vi "UserInput-String.vi"() -> ()   [LabVIEW 2019]
panel:
  in  "Clear Form":bool
  in  "Copy String":bool
  out "String Indicator - Output":string
  in  "String Control - Input":string
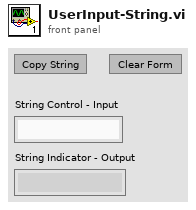
[diagram p1: front panel]
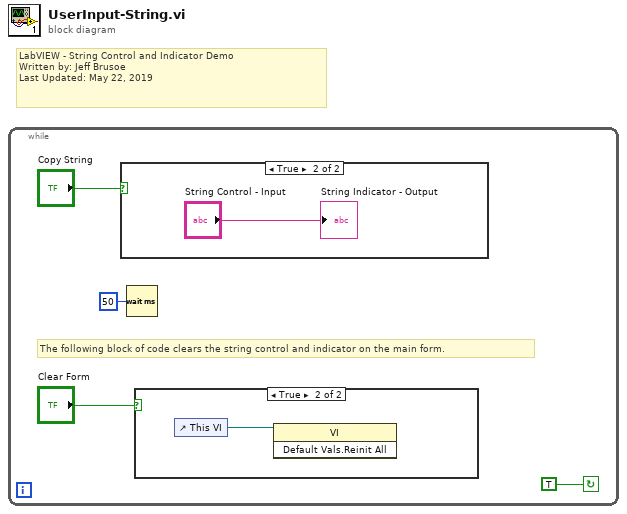
[diagram p0: block diagram]
diagram:
  # "LabVIEW - String Control and Indicator Demo\nWritten by: Jeff Brusoe\nLast Updated: May 22, 2019"
  n1 = while {
    stop <- TRUE continue-if-true
    # "The following block of code clears the string control and indicator on the main form."
    n2 = case shown="True" "Copy String" {
      frame False {
      }
      frame True {
        "String Indicator - Output" <- "String Control - Input"
      }
    }
    n3 = Wait (ms)(milliseconds to wait=u32 50) -> ()  [unwired: 1 out]
    n4 = case shown="True" "Clear Form" {
      frame False {
      }
      frame True {
        n5 = control-ref of="This VI"() -> (w5:refnum<vi>)
        n6 = invoke class="VI" method="Default Vals.Reinit All"(reference=w5) -> ()  [unwired: 2 in, 3 out]
      }
    }
  }
